vi "Swerve Rotation Math.vi"(9 "Wheel Speed":dbl, 10 "Wheel Angle":dbl, 11 "Encoder":dbl) -> (0 "Goal":dbl, 2 "Wheel Speed":dbl, 3 "Difference":dbl)   [LabVIEW 2023]
panel:
  # "Goal Angle"
  # "Input"
  # "Difference in degrees"
  # "Current Angle"
  # "Difference in Radians"
  # "Output"
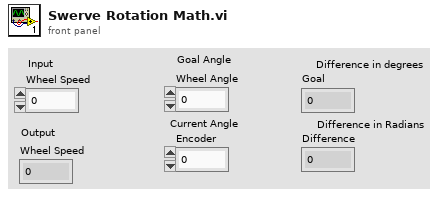
[diagram p1: front panel]
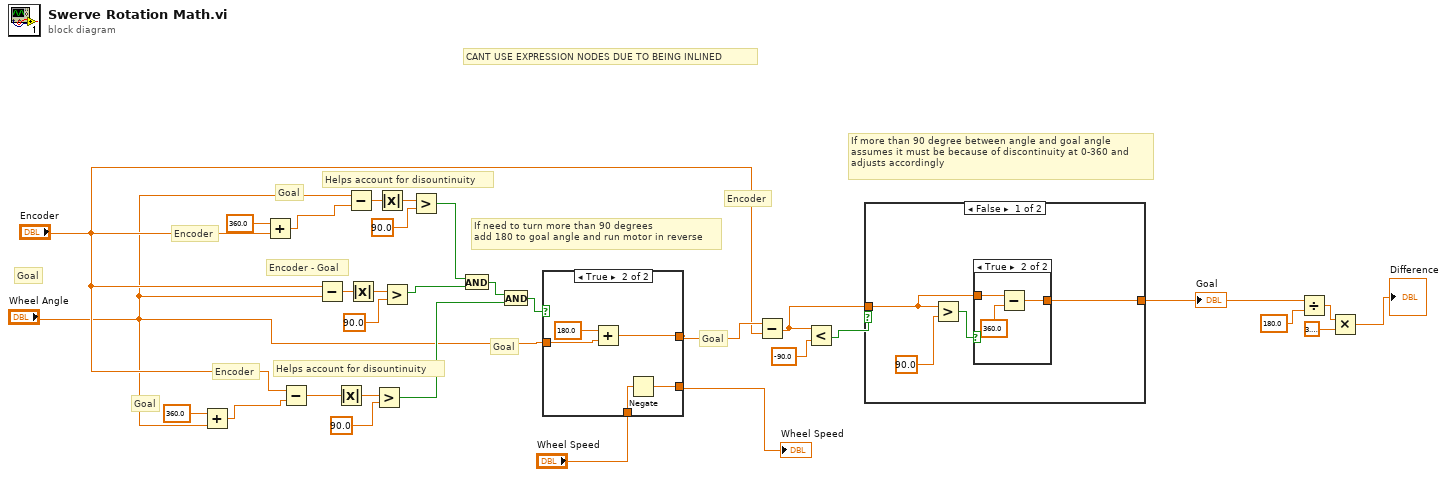
[diagram p0: block diagram]
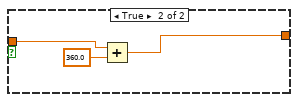
[diagram p3: hidden frame]
diagram:
  # "CANT USE EXPRESSION NODES DUE TO BEING INLINED"
  # "Helps account for disountinuity"
  # "Helps account for disountinuity"
  # "Encoder"
  # "Goal"
  # "Goal"
  # "Goal"
  # "Encoder"
  # "Goal"
  # "Goal"
  # "Encoder"
  # "Encoder - Goal"
  # "If more than 90 degree between angle and goal angle\nassumes it must be because of discontinuity at 0-360 and\nadjusts accordingly"
  # "If need to turn more than 90 degrees\nadd 180 to goal angle and run motor in reverse"
  n1 = Add(x=360.0, y="Wheel Angle") -> (x+y=w7:dbl)
  n2 = Add(x=360.0, y="Encoder") -> (x+y=w12:dbl)
  n3 = Subtract(x="Encoder", y=w7) -> (x-y=w30:dbl)
  n4 = Subtract(x="Encoder", y="Wheel Angle") -> (x-y=w25:dbl)
  n5 = Absolute Value(x=w30) -> (abs(x)=w29:dbl)
  n6 = Subtract(x="Wheel Angle", y=w12) -> (x-y=w31:dbl)
  n7 = Absolute Value(x=w25) -> (abs(x)=w24:dbl)
  n8 = Greater?(x=w29, y=90.0) -> (0:w21:bool)
  n9 = Absolute Value(x=w31) -> (abs(x)=w27:dbl)
  n10 = Greater?(x=w24, y=90.0) -> (0:w19:bool)
  n11 = Greater?(x=w27, y=90.0) -> (0:w18:bool)
  n12 = And(x=w18, y=w19) -> (x .and. y?=w20:bool)
  n13 = And(x=w20, y=w21) -> (x .and. y?=w22:bool)
  n14 = case shown="True" w22 {
    tunnel: "Wheel Angle" -> [w33 w38]
    tunnel: [w33 w36] -> w17
    tunnel: "Wheel Speed" -> [w32 w35]
    tunnel: [w32 w34] -> w8
    frame False {
    }
    frame True {
      n15 = Add(x=180.0, y=w38) -> (x+y=w36:dbl)
      n16 = Negate(x=w35) -> (-x=w34:dbl)
    }
  }
  "Wheel Speed" <- w8
  n17 = Subtract(x=w17, y="Encoder") -> (x-y=w14:dbl)
  n18 = Less?(x=w14, y=-90.0) -> (x < y?=w15:bool)
  n19 = case shown="False" w15 {
    tunnel: [w39 w48] -> w13
    tunnel: w14 -> [w40 w47]
    frame False {
      n20 = Greater?(x=w40, y=90.0) -> (0:w41:bool)
      n21 = case shown="True" w41 {
        tunnel: w40 -> [w43 w46]
        tunnel: [w43 w45] -> w39
        frame False {
        }
        frame True {
          n22 = Subtract(x=w46, y=360.0) -> (x-y=w45:dbl)
        }
      }
    }
    frame True {
      n23 = Add(x=w47, y=360.0) -> (x+y=w48:dbl)
    }
  }
  "Goal" <- w13
  n24 = Divide(x=w13, y=180.0) -> (x/y=w2:dbl)
  n25 = Multiply(x=w2, y=3.141592653589793) -> (x*y=→"Difference":dbl)
